vi "SerDes Configuration Script Example.vi"() -> ()   [LabVIEW 2023, in "GettingStarted_Common_148X_Host.lvlib"]
uses:
  GettingStarted_Common_148X_Host.lvlib
  <vilib>/userDefined/Silver/nirio_resource_slv.ctl
  <instrlib>/FlexRIO/Automotive Vision Utility/v1/Host/Types/TCP Socket Configuration.ctl
  <vilib>/FPGAPlugInAG/Dynamic/niLvFpga_Close_Dynamic.vi
  <vilib>/rvi/interface/nirviCloseFPGA/nirviCloseFPGA.xnode
  <instrlib>/FlexRIO/Automotive Vision Utility/v1/Host/Automotive Vision Utility.lvlib
panel:
  out "Running":bool
  out "error out":errorcluster
  in  "Process Stop Button":bool
  out "utility ouput":string caption="SerDes Configuration Utility Server Output"
  in  "Serial Channels":string[](array[string])
  in  "Configuration Script Path":path
  in  "RunScript Button":bool
  in  "Verbose":bool
  in  "Output File":path
  in  "TCP Socket Connection":T1={"host"="localhost", "port"=50505, "timeout"=10.0}
  in  "Bitfile Path":path
  in  "RIO Device":T2
  # "Overview: Execute serializer and deserializer configuration scripts.\nInstructions: \n 1. Select the RIO Device and corresponding Bitfile Path used to create and FPGA interface.\n 2. Update the SerDes Script Utility Server Configuration setttings or leave as default. This example makes use of an output file to display the results so if no Outfile File Path is chosen, a default location of SerDesConfigUtilLog.txt will be used.\n 3. Run the VI and wait for the Running LED to illuminate to indicate that the SerDes configuration utility is running.\n 4. Select the Serial Channels on which the configuration script will be run (i.e. \"SI0\" or \"SO0\").\n 5. Select the Configuration Script Path and click the Run Script button to execute the confiugration script on all selected serial channels.\n 6. Repeat steps 4 and 5 as desired.\n 7. Click the Close button to close the SerDes configuration utility and the FPGA interface."
  # "Resource Configuration"
  # "SerDes Script Utility Client Commands"
  # "SerDes Script Utiltiy Server Configuration"
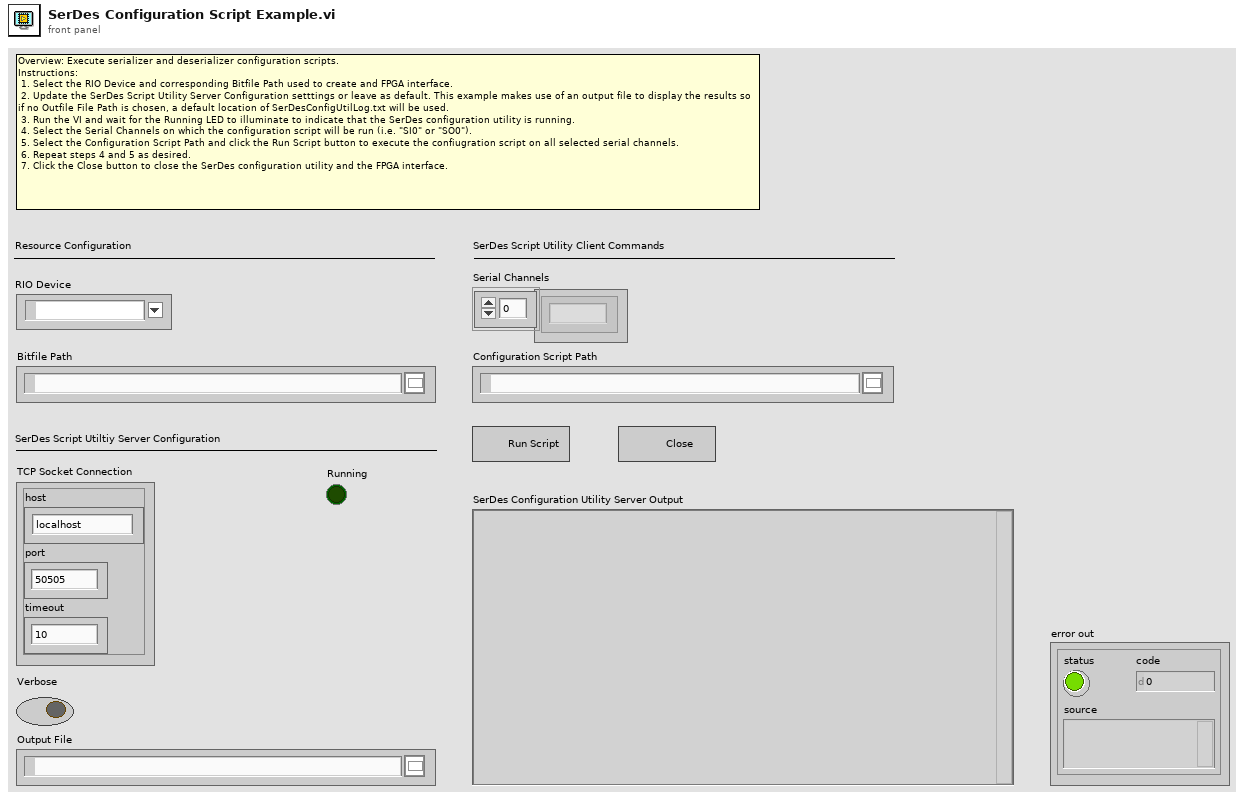
[diagram p1: front panel]
types:
  T1 = typedef "Automotive Vision Utility.lvlib/TCP Socket Configuration.ctl" = cluster{"host":string, "port":u16, "timeout":dbl}
  T2 = typedef "nirio_resource_slv.ctl" = tag
  T3 = enum16{"open", "replace", "create", "open or create", "replace or create", "replace or create with confirmation"}
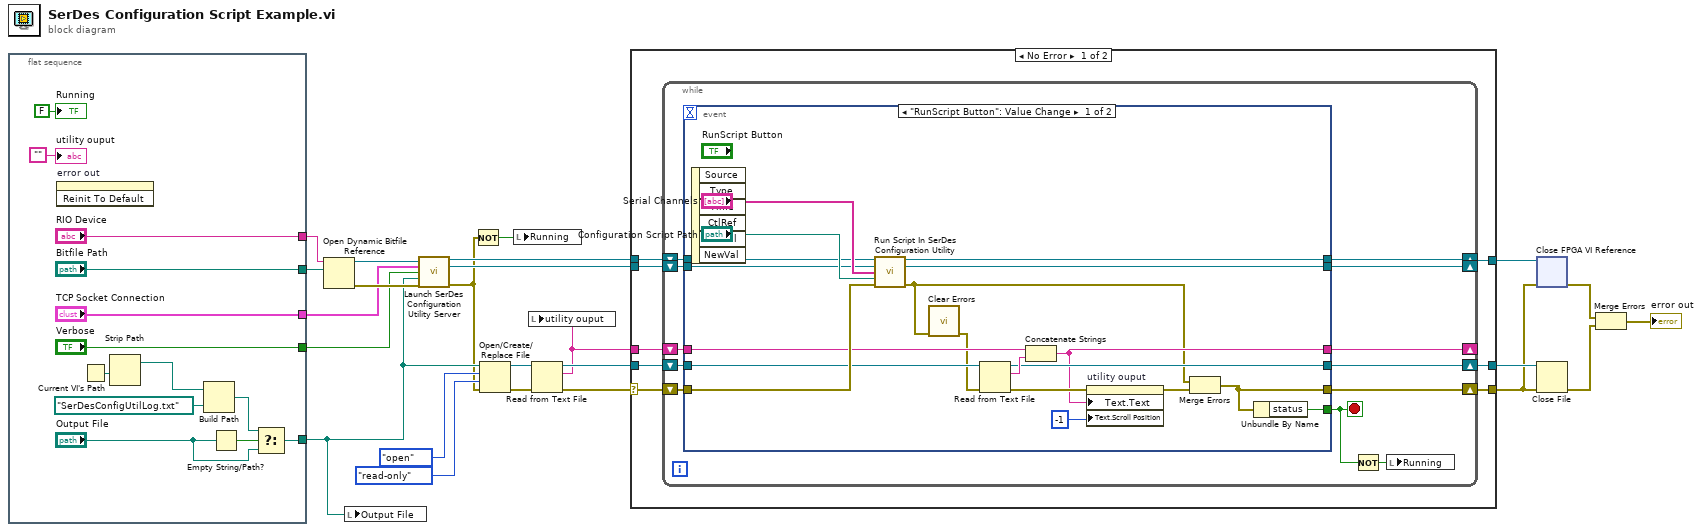
[diagram p0: block diagram]
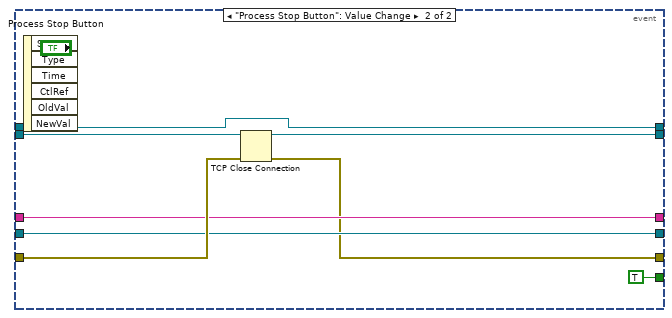
[diagram p2: hidden frame]
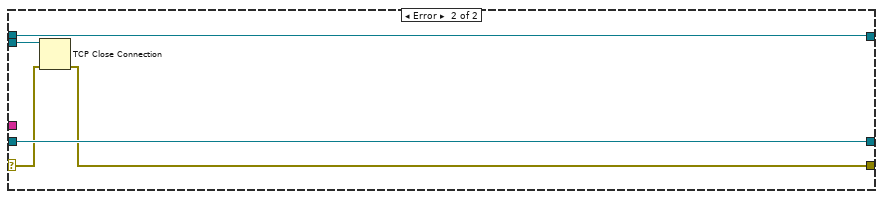
[diagram p3: hidden frame]
diagram:
  n1 = flat-sequence {
    tunnel: ["RIO Device"] -> w7
    tunnel: ["Bitfile Path"] -> w23
    tunnel: ["Verbose"] -> w20
    tunnel: ["TCP Socket Connection"] -> w19
    tunnel: [w26] -> w5
    frame #0 {
      n2 = invoke on="error out" class="Clust (strict)" method="Reinit To Default"() -> ()  [unwired: 3 in, 3 out]
      n3 = Current VI's Path() -> (path=w25:path)
      n4 = Strip Path(path=w25) -> (stripped path=w24:path)  [unwired: 1 out]
      n5 = Build Path(base path=w24, name or relative path=path "SerDesConfigUtilLog.txt") -> (appended path=w27:path)
      n6 = Empty String/Path?(string/path="Output File") -> (empty?=w29:bool)
      n7 = Select(t=w27, s=w29, f="Output File") -> (s? t:f=w26:path)
      "Running" <- FALSE ("Running")
      "utility ouput" <- ""
    }
  }
  n8 = Open Dynamic Bitfile Reference(0:w7, 1:w23) -> (5:w21:refnum<k20>, 8:w22:errorcluster)  [unwired: 3 in]
  n9 = local write "Output File"(w5) -> ()
  n10 = call <instrlib>:"Launch SerDes Configuration Utility Server.vi"("fpga interface in"=w21, "tcp socket config"=w19, "verbose (F)"=w20, "output file"=w5, "error in"=w22) -> ("fpga interface out"=w15:refnum<k20>, "socket connection id out"=w14:refnum<k5>, "error out"=w4:errorcluster)  [unwired: 8 in]
  n11 = Not(x=w4) -> (.not. x?=w6:bool)
  n12 = Open/Create/Replace File(file path (use dialog)=w5, error in=w4, operation (0:open)=T3."open", access (0:read/write)=enum16{"read/write", "read-only", "write-only"}."read-only") -> (refnum out=w16:refnum<file>, error out=w2:errorcluster)  [unwired: 2 in, 1 out]
  n13 = local write "Running"(w6) -> ()
  n14 = Read from Text File(file (use dialog)=w16, error in=w2) -> (text=w3:string, error out=w1:errorcluster)  [unwired: 2 in, 2 out]
  n15 = local write "utility ouput"(w3) -> ()
  n16 = case shown="No Error" w1 {
    selector: w1 -> [w37 w84]
    tunnel: w16 -> [w39 w87]
    tunnel: w15 -> [w44 w88]
    tunnel: w14 -> [w43 w86]
    tunnel: [w42 w87] -> w13
    tunnel: [w41 w88] -> w12
    tunnel: [w40 w85] -> w8
    tunnel: w3 -> [w38 _]
    frame No Error {
      n17 = while {
        shift-right: [w51] -> w40
        shift-left: w37 -> [w56]
        shift-right: [w52] -> w42
        shift-left: w39 -> [w55]
        shift-right: [w53] -> _
        shift-left: w38 -> [w54]
        shift-right: [w48] -> w41
        shift-left: w44 -> [w50]
        shift-right: [w47] -> _
        shift-left: w43 -> [w49]
        stop <- w45 stop-if-true
        n18 = event shown="[0] \"RunScript Button\": Value Change" {
          selector: _ -> [_ _]
          dyn-events: _ -> [_ _]
          timeout: _ -> [_ _]
          tunnel: w56 -> [w73 w82]
          tunnel: w55 -> [w72 w77]
          tunnel: w54 -> [w71 w78]
          tunnel: [w61 w78] -> w53
          tunnel: [w69 w77] -> w52
          tunnel: [w59 w76] -> w51
          tunnel: w50 -> [w68 w80]
          tunnel: w49 -> [w67 w83]
          tunnel: [w66 w80] -> w48
          tunnel: [w65 w81] -> w47
          tunnel: [w64 TRUE] -> w45
          event "RunScript Button": Value Change {
            n19 = event-data() -> ()  [unwired: 1 in, 6 out]
            n20 = call <instrlib>:"Run Script In SerDes Configuration Utility.vi"("fpga interface in"=w68, "socket connection id in"=w67, "serial channels"="Serial Channels", "configuration script"="Configuration Script Path", "error in"=w73) -> ("fpga interface out"=w66:refnum<k20>, "socket connection id out"=w65:refnum<k5>, "error out"=w58:errorcluster)  [unwired: 8 in]
            n21 = call <vilib>:"Clear Errors.vi"("error in (no error)"=w58) -> ("error out"=w57:errorcluster)  [unwired: 5 in, 1 out]
            n22 = Read from Text File(file (use dialog)=w72, error in=w57) -> (refnum out=w69:refnum<file>, text=w70:string, error out=w63:errorcluster)  [unwired: 2 in, 1 out]
            n23 = Concatenate Strings(w71, w70) -> (w61:string)
            n24 = property on="utility ouput" class="Str"(error in=w63, "Text.Text"=w61, "Text.Scroll Position"=-1) -> (error out=w60:errorcluster)  [unwired: 1 in, 1 out]
            n25 = Merge Errors(w58, w60) -> (w59:errorcluster)
            n26 = Unbundle By Name(w59) -> ("status"=w64:bool)
          }
          event "Process Stop Button": Value Change {
            n27 = event-data() -> ()  [unwired: 1 in, 6 out]
            n28 = TCP Close Connection(connection ID=w83, error in (no error)=w82) -> (connection ID out=w81:refnum<k5>, error out=w76:errorcluster)  [unwired: 1 in]
          }
        }
        n29 = Not(x=w45) -> (.not. x?=w46:bool)
        n30 = local write "Running"(w46) -> ()
      }
    }
    frame Error {
      n31 = TCP Close Connection(connection ID=w86, error in (no error)=w84) -> (error out=w85:errorcluster)  [unwired: 1 in, 1 out]
    }
  }
  n32 = xnode "Close FPGA VI Reference"("FPGA VI Reference In"=w12, "error in"=w8) -> ("error out"=w11:errorcluster)
  n33 = Close File(refnum=w13, error in=w8) -> (error out=w10:errorcluster)  [unwired: 1 out]
  n34 = Merge Errors(w11, w10) -> (→"error out":errorcluster)
